vi "Send Has Destroyed.vi"(8 "Error in":errorcluster, 10 "Actor":refnum<class "Actor.lvclass">) -> ()   [LabVIEW 2020, in "jettl.lvlib" / "Actor.lvlib"]
uses:
  Actor.lvlib
  Actor/Actor.lvclass
  Has Destroyed Msg/Has Destroyed Msg.lvlib
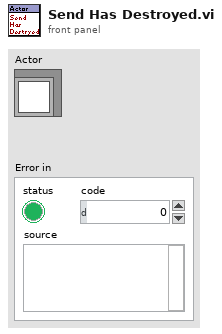
[diagram p1: front panel]
types:
  T1 = typedef "jettl.lvlib/Actor.lvlib/Created Aliases.ctl" = set{string}
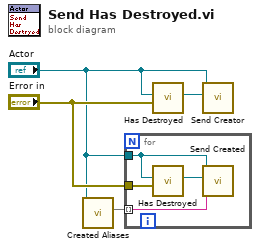
[diagram p0: block diagram]
diagram:
  n1 = call-dynamic "Created Aliases.vi"("Actor in"="Actor") -> ("Created Aliases"=w4:T1)  [unwired: 10 in]
  n2 = for {
    tunnel: "Actor" -> [w7]
    tunnel: w4 -> [w8] mode=indexing
    tunnel: "Error in" -> [w5]
    n3 = call "Has Destroyed.vi"("Error"=w5, "Actor"=w7) -> ("Msg"=w6:refnum<class "Msg.lvclass">)  [unwired: 9 in]
    n4 = call-dynamic "Send Created.vi"("Alias"=w8, "Msg"=w6, "Actor in"=w7) -> ()  [unwired: 8 in, 1 out]
  }
  n5 = call "Has Destroyed.vi"("Error"="Error in", "Actor"="Actor") -> ("Msg"=w3:refnum<class "Msg.lvclass">)  [unwired: 9 in]
  n6 = call-dynamic "Send Creator.vi"("Msg"=w3, "Actor in"="Actor") -> ()  [unwired: 9 in, 1 out]
